vi "ConversionFORCEGLD.vi"(0 "Accel (Dyna LF)":dbl, 1 "Accel (Dyna LF) Offset":dbl, 2 "grams (Omega GF)":dbl, 3 "grams (Omega GF) Offset":dbl, 4 "Futek  (Static LF)":dbl, 5 "Futek  (Static LF) Offset":dbl, 7 "Weight added (kg)":dbl) -> (15 "Dyna LF [N]":dbl, 17 "GF [N]":dbl, 19 "Static LF [N]":dbl)   [LabVIEW 2020]
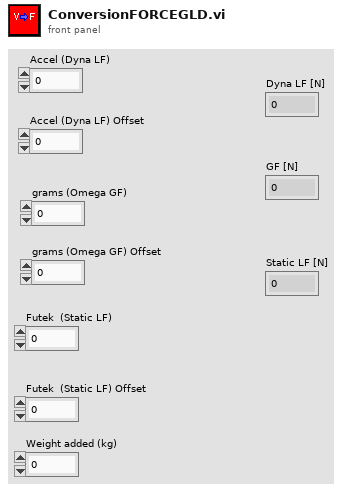
[diagram p1: front panel]
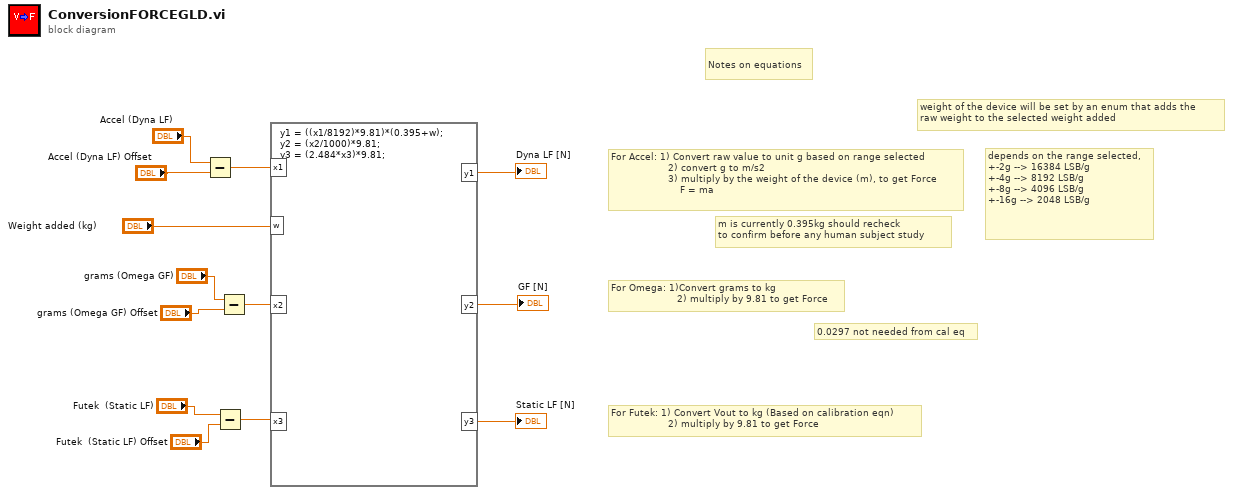
[diagram p0: block diagram]
diagram:
  # "0.0297 not needed from cal eq"
  # "m is currently 0.395kg should recheck\nto confirm before any human subject study"
  # "weight of the device will be set by an enum that adds the \nraw weight to the selected weight added"
  # "For Futek: 1) Convert Vout to kg (Based on calibration eqn)\n                   2) multiply by 9.81 to get Force"
  # "For Omega: 1)Convert grams to kg \n                      2) multiply by 9.81 to get Force"
  # "For Accel: 1) Convert raw value to unit g based on range selected\n                   2) convert g to m/s2 \n                   3) multiply by the weight of the device (m), to get Force\n                       F = ma"
  # "depends on the range selected,\n+-2g --> 16384 LSB/g\n+-4g --> 8192 LSB/g\n+-8g --> 4096 LSB/g\n+-16g --> 2048 LSB/g"
  # "Notes on equations"
  n1 = Subtract(x="Accel (Dyna LF)", y="Accel (Dyna LF) Offset") -> (x-y=w4:dbl)
  n2 = Subtract(x="Futek  (Static LF)", y="Futek  (Static LF) Offset") -> (x-y=w2:dbl)
  n3 = Subtract(x="grams (Omega GF)", y="grams (Omega GF) Offset") -> (x-y=w3:dbl)
  n4 = formula code="y1 = ((x1/8192)*9.81)*(0.395+w);\ny2 = (x2/1000)*9.81;\ny3 = (2.484*x3)*9.81;"("x1"=w4, "x2"=w3, "x3"=w2, "w"="Weight added (kg)") -> ("y2"=→"GF [N]":dbl, "y1"=→"Dyna LF [N]":dbl, "y3"=→"Static LF [N]":dbl)
